vi "BlinkTest.vi"() -> ()   [LabVIEW 2019]
panel:
  in  "VISA":refnum<visa-resource-name>
  out "Console":string
  in  "code":string="/*\n  Blink\n\n  Turns an LED on for one second, then off for one second, repeatedly.\n\n  Most Arduinos have an on-board LED you can control. On the UNO, MEGA and ZERO\n  it is attached to digital pin 13, on MKR1000 on pin 6. LED_BUILTIN is set to\n  the correct LED pin independent of which board is used.\n  If you want to know what pin the on-board LED is connected to on your Arduino\n  model, check the Technical Specs of your board at:\n  https://www.arduino.cc/en/Main/Products\n\n  modified 8 May 2014\n  by Scott Fitzgerald\n  modified 2 Sep 2016\n  by Arturo Guadalupi\n  modified 8 Sep 2016\n  by Colby Newman\n\n  This example code is in the public domain.\n\n  http://www.arduino.cc/en/Tutorial/Blink\n*/\n\n// the setup function runs once when you press reset or power the board\nvoid setup() {\n  // initialize digital pin LED_BUILTIN as an output.\n  pinMode(LED_BUILTIN, OUTPUT);\n}\n\n// the loop function runs over and over again forever\nvoid loop() {\n  digitalWrite(LED_BUILTIN, HIGH);   // turn the LED on (HIGH is the voltage level)\n  delay(1000);                       // wait for a second\n  digitalWrite(LED_BUILTIN, LOW);    // turn the LED off by making the voltage LOW\n  delay(1000);                       // wait for a second\n}"
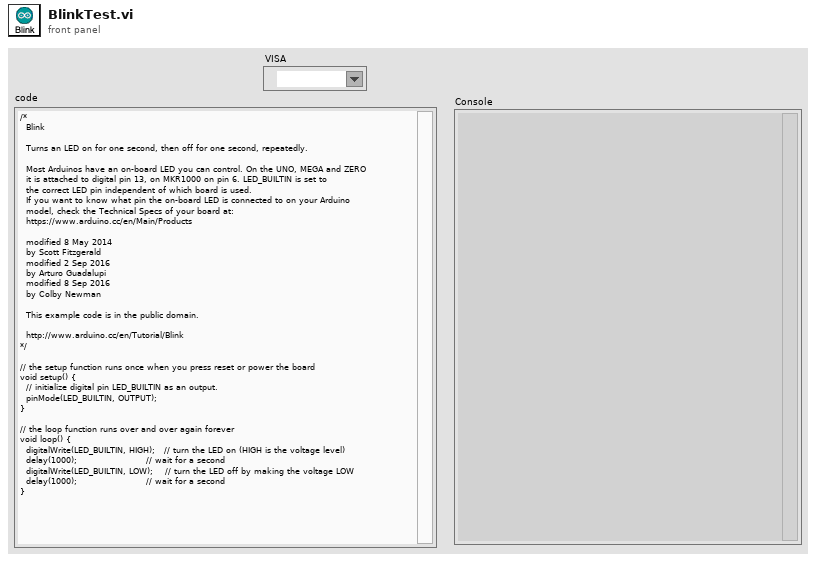
[diagram p1: front panel]
types:
  T1 = typedef "Arduino.ctl" = cluster{"Java":path, "Packages":path, "folder":path, "serial":string, "Console":string}
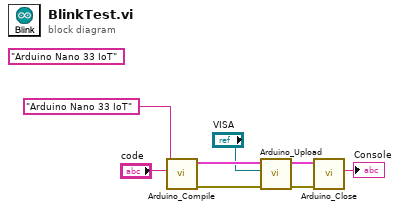
[diagram p0: block diagram]
diagram:
  (unwired) "Arduino Nano 33 IoT" ("Board")
  n1 = call <userlib>:"Arduino_Compile.vi"("Code"="code", "Board"="Arduino Nano 33 IoT") -> ("error out"=w8:errorcluster, "Arduino Out"=w6:T1)  [unwired: 8 in]
  n2 = call <userlib>:"Arduino_Upload.vi"("error in (no error)"=w8, "VISA resource name"="VISA", "Arduino In"=w6) -> ("error out"=w7:errorcluster, "Arduino Out"=w5:T1)  [unwired: 7 in]
  n3 = call <userlib>:"Arduino_Close.vi"("error in (no error)"=w7, "Arduino In"=w5) -> ("Console"=→"Console":string)  [unwired: 8 in, 1 out]
